vi "DN4_AO_InstantWrite.vi"(2 "error in (no error)":errorcluster, 3 "Dynamic Data Type":dynamicdata(waveform), 4 "Task ID":u32) -> (0 "error out":errorcluster, 1 "Task ID":u32)   [LabVIEW 2009]
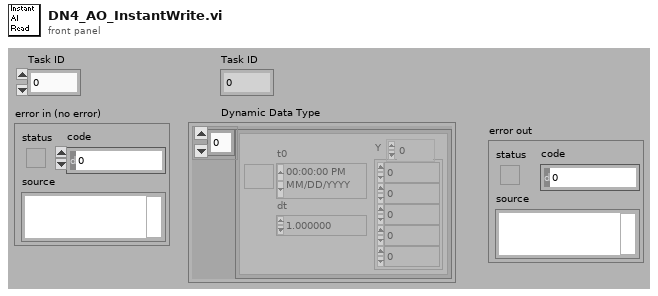
[diagram p1: front panel]
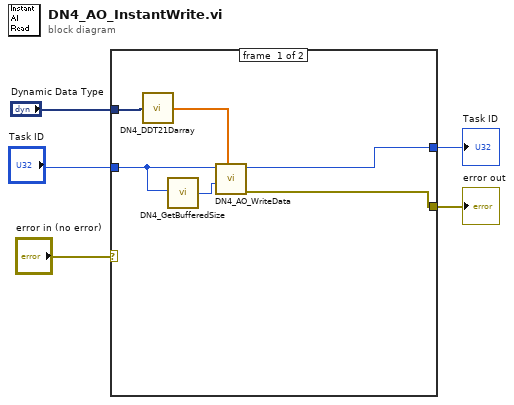
[diagram p0: block diagram]
diagram:
  n1 = case shown="No Error" "error in (no error)" {
    selector: "error in (no error)" -> [_ w12]
    tunnel: "Task ID" -> [w7 w13]
    tunnel: [w9 w12] -> w4
    tunnel: [w8 w13] -> w3
    tunnel: "Dynamic Data Type" -> [w11 _]
    frame #0 {
      n2 = call <userlib>:"DN4_DDT21Darray.vi"("data"=w11) -> ("Array"=w10:dbl[])
      n3 = call <userlib>:"DN4_GetBufferedSize.vi"("Task ID"=w7) -> ("return type"=w6:i32)
      n4 = call <userlib>:"DN4_AO_WriteData.vi"("data"=w10, "count"=w6, "Task ID"=w7) -> ("error out"=w9:errorcluster, "Task ID"=w8:u32)  [unwired: 2 in, 5 out]
    }
    frame #1 {
    }
  }
  "error out" <- w4
  "Task ID" <- w3
